vi "6-15.vi"() -> ()   [LabVIEW 2017]
panel:
  out "Waveform Chart":dbl(graph)
  in  "Stop Button":bool
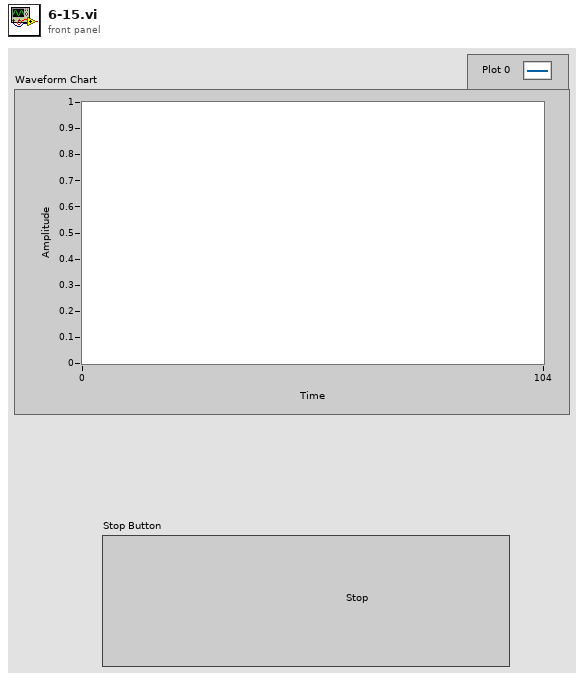
[diagram p1: front panel]
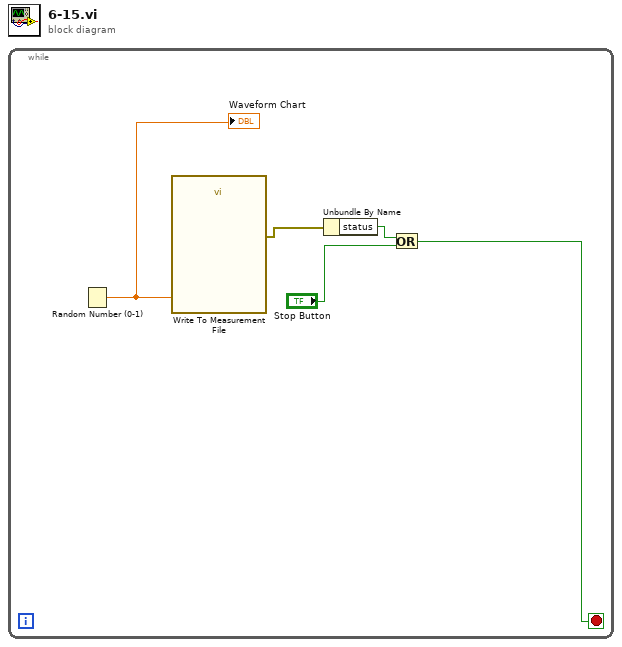
[diagram p0: block diagram]
diagram:
  n1 = while {
    stop <- w4 stop-if-true
    n2 = Random Number (0-1)() -> (number: 0 to 1=w1:dbl)
    "Waveform Chart" <- w1
    n3 = call "Write To Measurement File"("Signals"=w1) -> ("error out"=w3:errorcluster)  [unwired: 16 in, 2 out]
    n4 = Unbundle By Name(w3) -> ("status"=w2:bool)
    n5 = Or(x=w2, y="Stop Button") -> (x .or. y?=w4:bool)
  }
